vi "Configure External Logging Trigger Source.vi"(8 "error in (no error)":errorcluster, 10 "External Logging Trigger Source (0: Bus)":u16(ring) items=["Bus", "External", "Immediate", "Pin 1", "Pin 2", "Pin 3", "Pin 4", "Pin 5", "Pin 6", "Pin 7"], 11 "VISA resource name":refnum<visa-resource-name>) -> (0 "error out":errorcluster, 3 "VISA resource name out":refnum<visa-resource-name>)   [LabVIEW 2021, in "Agilent N6900 N7900 Series.lvlib"]
doc: "Selects the trigger source forthe External Logging system"
uses:
  <instrlib>/Agilent N6900 N7900 Series/Agilent N6900 N7900 Series.lvlib
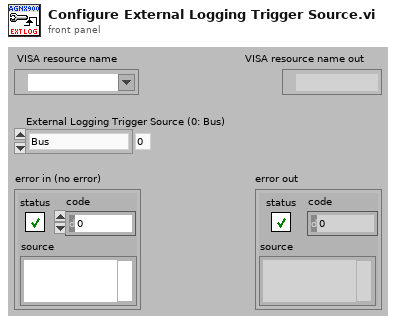
[diagram p1: front panel]
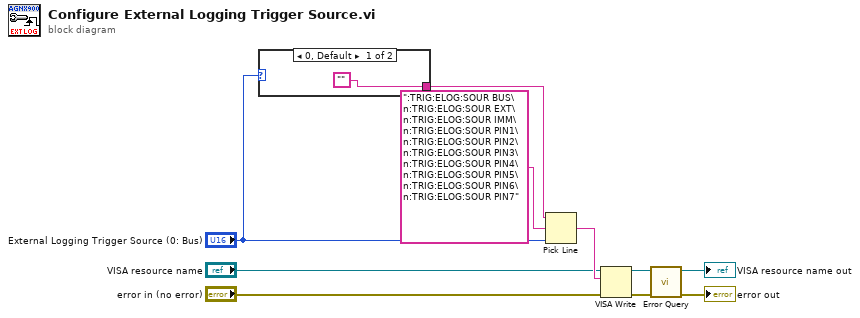
[diagram p0: block diagram]
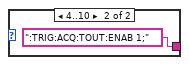
[diagram p2: hidden frame]
diagram:
  n1 = case shown="0, Default" "External Logging Trigger Source (0: Bus)" {
    tunnel: ["" ("string (\"\")") ":TRIG:ACQ:TOUT:ENAB 1;" ("string (\"\")")] -> w9
    frame 0, Default {
    }
    frame 4..10 {
    }
  }
  n2 = Pick Line(string ("")=w9, multi-line string=":TRIG:ELOG:SOUR BUS\n:TRIG:ELOG:SOUR EXT\n:TRIG:ELOG:SOUR IMM\n:TRIG:ELOG:SOUR PIN1\n:TRIG:ELOG:SOUR PIN2\n:TRIG:ELOG:SOUR PIN3\n:TRIG:ELOG:SOUR PIN4\n:TRIG:ELOG:SOUR PIN5\n:TRIG:ELOG:SOUR PIN6\n:TRIG:ELOG:SOUR PIN7", line index="External Logging Trigger Source (0: Bus)") -> (output string=w8:string)
  n3 = VISA Write(VISA resource name="VISA resource name", write buffer=w8, error in (no error)="error in (no error)") -> (VISA resource name out=w5:refnum<visa-resource-name>, error out=w4:errorcluster)  [unwired: 1 out]
  n4 = call <instrlib>:"Error Query.vi"("error in (no error)"=w4, "VISA resource name"=w5) -> ("error out"=→"error out":errorcluster, "VISA resource name out"=→"VISA resource name out":refnum<visa-resource-name>)  [unwired: 6 in, 2 out]
